vi "Register API.vi"(8 "error in (no error)":errorcluster, 10 "API":refnum<class "API.lvclass">, 11 "VolatusAPI in":refnum<class "VolatusAPI.lvclass">) -> (0 "error out":errorcluster, 3 "VolatusAPI out":refnum<class "VolatusAPI.lvclass">)   [LabVIEW 2020, in "Volatus.lvlib" / "VolatusAPI.lvclass"]
uses:
  VolatusAPI.lvclass
  VolatusAPI.lvclass/VolatusAPI.ctl
  Identity/Identity.lvclass
  API/API.lvclass
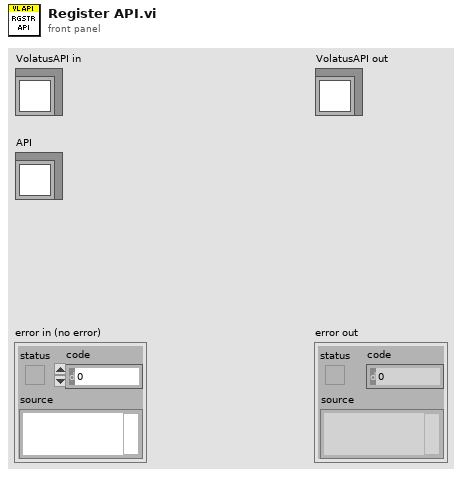
[diagram p1: front panel]
types:
  T1 = typedef "Volatus.lvlib/VolatusAPI.lvclass/APIs Ref.ctl" = cluster{"API Numbers":map{string, u32}, "APIs":map{u32, refnum<class "API.lvclass">}, "Next API":u32}
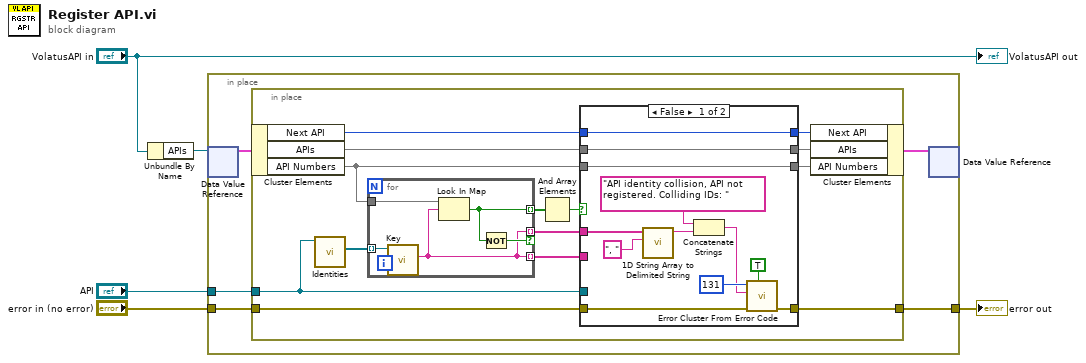
[diagram p0: block diagram]
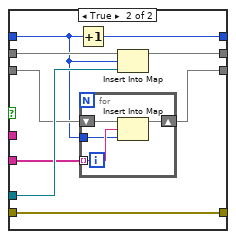
[diagram p2: hidden frame]
diagram:
  n1 = Unbundle By Name("VolatusAPI in") -> ("APIs"=w2:refnum<data-value>)
  n2 = in-place {
    in-place-border: "API" -> [w10]
    in-place-border: "error in (no error)" -> [w9]
    in-place-border: [w6] -> w1
    n3 = in-place-dvr #1(w2) -> (w8:T1)  [unwired: 1 out]
    n4 = in-place {
      in-place-border: w10 -> [w19]
      in-place-border: w9 -> [w18]
      in-place-border: [w11] -> w6
      n5 = in-place-cluster #2(w8) -> ("Next API"=w13:u32, "APIs"=w16:map{u32, refnum<class "API.lvclass">}, "API Numbers"=w17:map{string, u32})
      n6 = call-dynamic "Identities.vi"("API in"=w19) -> ("Identities"=w24:refnum<class "Identity.lvclass">[])  [unwired: 8 in, 2 out]
      n7 = for {
        tunnel: w24 -> [w53] mode=indexing
        tunnel: w17 -> [w54]
        tunnel: [w52] -> w23 mode=indexing
        tunnel: [w50] -> w21 mode=indexing if=w51
        tunnel: [w50] -> w20 mode=indexing
        n8 = call "Key.vi"("Identity in"=w53) -> ("Key"=w50:string)  [unwired: 10 in]
        n9 = Look In Map(map=w54, key=w50) -> (key not found?=w52:bool)  [unwired: 1 in, 1 out]
        n10 = Not(x=w52) -> (.not. x?=w51:bool)
      }
      n11 = And Array Elements(Boolean array=w23) -> (logical AND=w22:bool)
      n12 = case shown="False" w22 {
        tunnel: w17 -> [w28 w42]
        tunnel: w18 -> [w36 w41]
        tunnel: w21 -> [w35 _]
        tunnel: [w29 w41] -> w11
        tunnel: w20 -> [_ w43]
        tunnel: w16 -> [w27 w45]
        tunnel: w19 -> [_ w44]
        tunnel: [w28 w40] -> w15
        tunnel: [w27 w39] -> w14
        tunnel: w13 -> [w26 w38]
        tunnel: [w26 w37] -> w12
        frame False {
          n13 = call <vilib>:"1D String Array to Delimited String.vi"("delimiter"=", ", "string array"=w35) -> ("delimited string"=w32:string)  [unwired: 9 in]
          n14 = Concatenate Strings("API identity collision, API not registered. Colliding IDs: ", w32) -> (w30:string)
          n15 = call <vilib>:"Error Cluster From Error Code.vi"("show call chain? (False)"=TRUE, "error in (no error)"=w36, "error message (\"\")"=w30, "error code (0)"=131) -> ("error out"=w29:errorcluster)  [unwired: 5 in]
        }
        frame True {
          n16 = Increment(x=w38) -> (x+1=w37:u32)
          n17 = for {
            tunnel: w43 -> [w47] mode=indexing
            shift-right: [w48] -> w40
            shift-left: w42 -> [w49]
            tunnel: w38 -> [w46]
            n18 = Insert Into Map(map in=w49, key=w47, value=w46) -> (map out=w48:map{string, u32})  [unwired: 2 out]
          }
          n19 = Insert Into Map(map in=w45, key=w38, value=w44) -> (map out=w39:map{u32, refnum<class "API.lvclass">})  [unwired: 2 out]
        }
      }
      n20 = in-place-cluster #2("Next API"=w12, "APIs"=w14, "API Numbers"=w15) -> (w7:T1)
    }
    n21 = in-place-dvr #1(w7) -> ()  [unwired: 2 out]
  }
  "error out" <- w1
  "VolatusAPI out" <- "VolatusAPI in"
